vi "Fit.vi"(8 "error in (no error)":errorcluster caption="entrée d'erreur (pas d'erreur)", 9 "doc":string, 10 "X":string[][](array[string]), 11 "HashingVectorizer.lvclass 2":refnum<class "HashingVectorizer.lvclass">) -> (0 "error out":errorcluster caption="sortie d'erreur", 2 "String Data":string, 3 "HashingVectorizer.lvclass":refnum<class "HashingVectorizer.lvclass">)   [LabVIEW 2020, in "HashingVectorizer.lvclass"]
doc: "Transform a sequence of documents to a document-term matrix.\n\nReturns :\n\n- String : OK"
uses:
  HashingVectorizer.lvclass
  HashingVectorizer.lvclass/HashingVectorizer.ctl
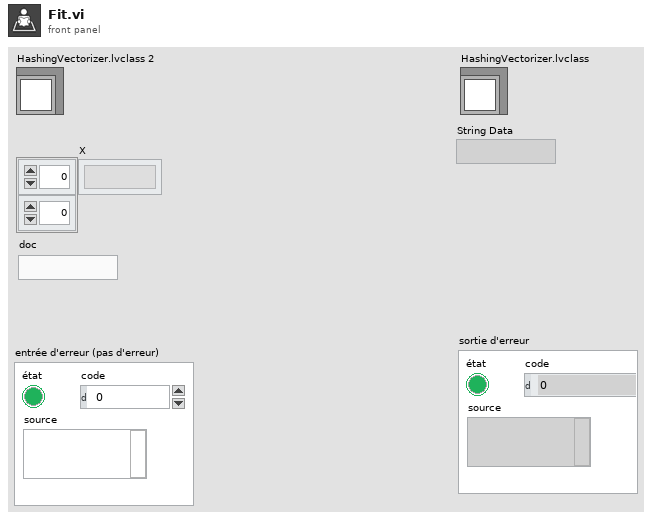
[diagram p1: front panel]
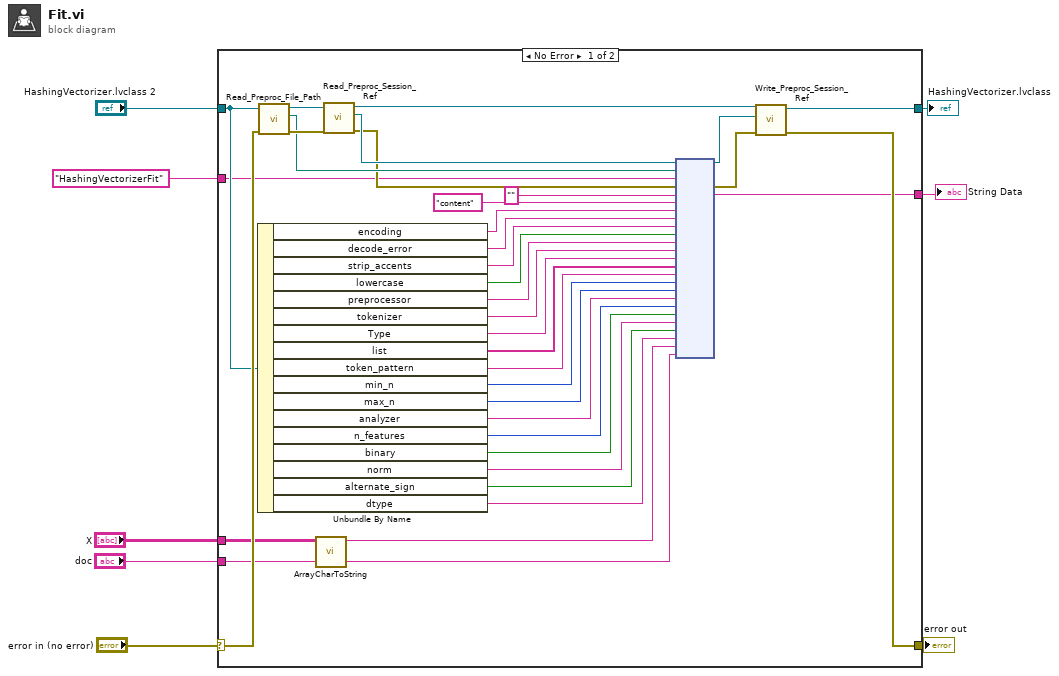
[diagram p0: block diagram]
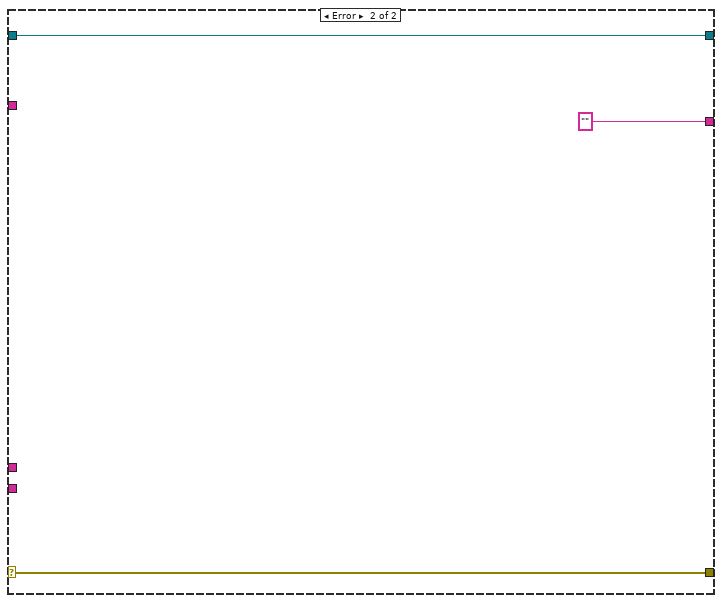
[diagram p2: hidden frame]
diagram:
  n1 = case shown="No Error" "error in (no error)" {
    selector: "error in (no error)" -> [w32 w47]
    tunnel: [w33 w47] -> w7
    tunnel: [w9 w46] -> w5
    tunnel: "HashingVectorizer.lvclass 2" -> [w31 w46]
    tunnel: "HashingVectorizerFit" ("Fonction") -> [w30 _]
    tunnel: [w24 ""] -> w3
    tunnel: "X" -> [w11 _]
    tunnel: "doc" -> [w12 _]
    frame No Error {
      n2 = Unbundle By Name(w31) -> ("encoding"=w35:string, "decode_error"=w34:string, "strip_accents"=w29:string, "lowercase"=w28:bool, "preprocessor"=w27:string, "tokenizer"=w26:string, "Type"=w23:string, "list"=w22:string[], "token_pattern"=w21:string, "min_n"=w20:i32, "max_n"=w19:i32, "analyzer"=w18:string, "n_features"=w17:i32, "binary"=w16:bool, "norm"=w15:string, "alternate_sign"=w14:bool, "dtype"=w13:string)
      n3 = call-dynamic "Read_Preproc_File_Path.vi"("error in (no error)"=w32, "Python in"=w31) -> ("error out"=w43:errorcluster, "File_Path"=w42:path, "Python out"=w44:refnum<class "HashingVectorizer.lvclass">)  [unwired: 7 in]
      n4 = call "ArrayCharToString.vi"("TAB"=w11) -> ("Instruction"=w10:string)  [unwired: 10 in]
      n5 = call-dynamic "Read_Preproc_Session_Ref.vi"("error in (no error)"=w43, "Python in"=w44) -> ("error out"=w40:errorcluster, "Session_ref"=w41:refnum<k35>, "Python out"=w39:refnum<class "HashingVectorizer.lvclass">)  [unwired: 7 in]
      n6 = node(w41, w42, w30, w40, "", "content", w35, w34, w29, w28, w27, w26, w23, w22, w21, w20, w19, w18, w17, w16, w15, w14, w13, w10, w12) -> (w37:refnum<k35>, w38:errorcluster, w24:string)  [unwired: 20 in, 2 out]
      n7 = call-dynamic "Write_Preproc_Session_Ref.vi"("error in (no error)"=w38, "Session_ref"=w37, "Python in"=w39) -> ("error out"=w33:errorcluster, "Python out"=w9:refnum<class "HashingVectorizer.lvclass">)  [unwired: 7 in]
    }
    frame Error {
    }
  }
  "error out" <- w7
  "HashingVectorizer.lvclass" <- w5
  "String Data" <- w3
